vi "Логи_Флаги.vi"() -> ()   [LabVIEW 2013]
panel:
  in  "Tab Control":T1(tab)
  out "?":cluster{dbl[], u16[]}[](graph)
  out "XY":cluster{dbl[], dbl[]}[](graph)
  out "double precision float":dbl
  out "ID параметров":u8[](array[numeric])
  out "Заголовок":string
  out "Количество параметров":u8
  out "size (in bytes)":i64
  # "1-VALUE_TRANSMITTED\n2-VOLTAGE_LOW\n3-FAIL_SENSOR\t\n4-ARMING_DISARMING\n5-FLAG_FAIL_SD\n6-FLAG_LIFT_COMMAND"
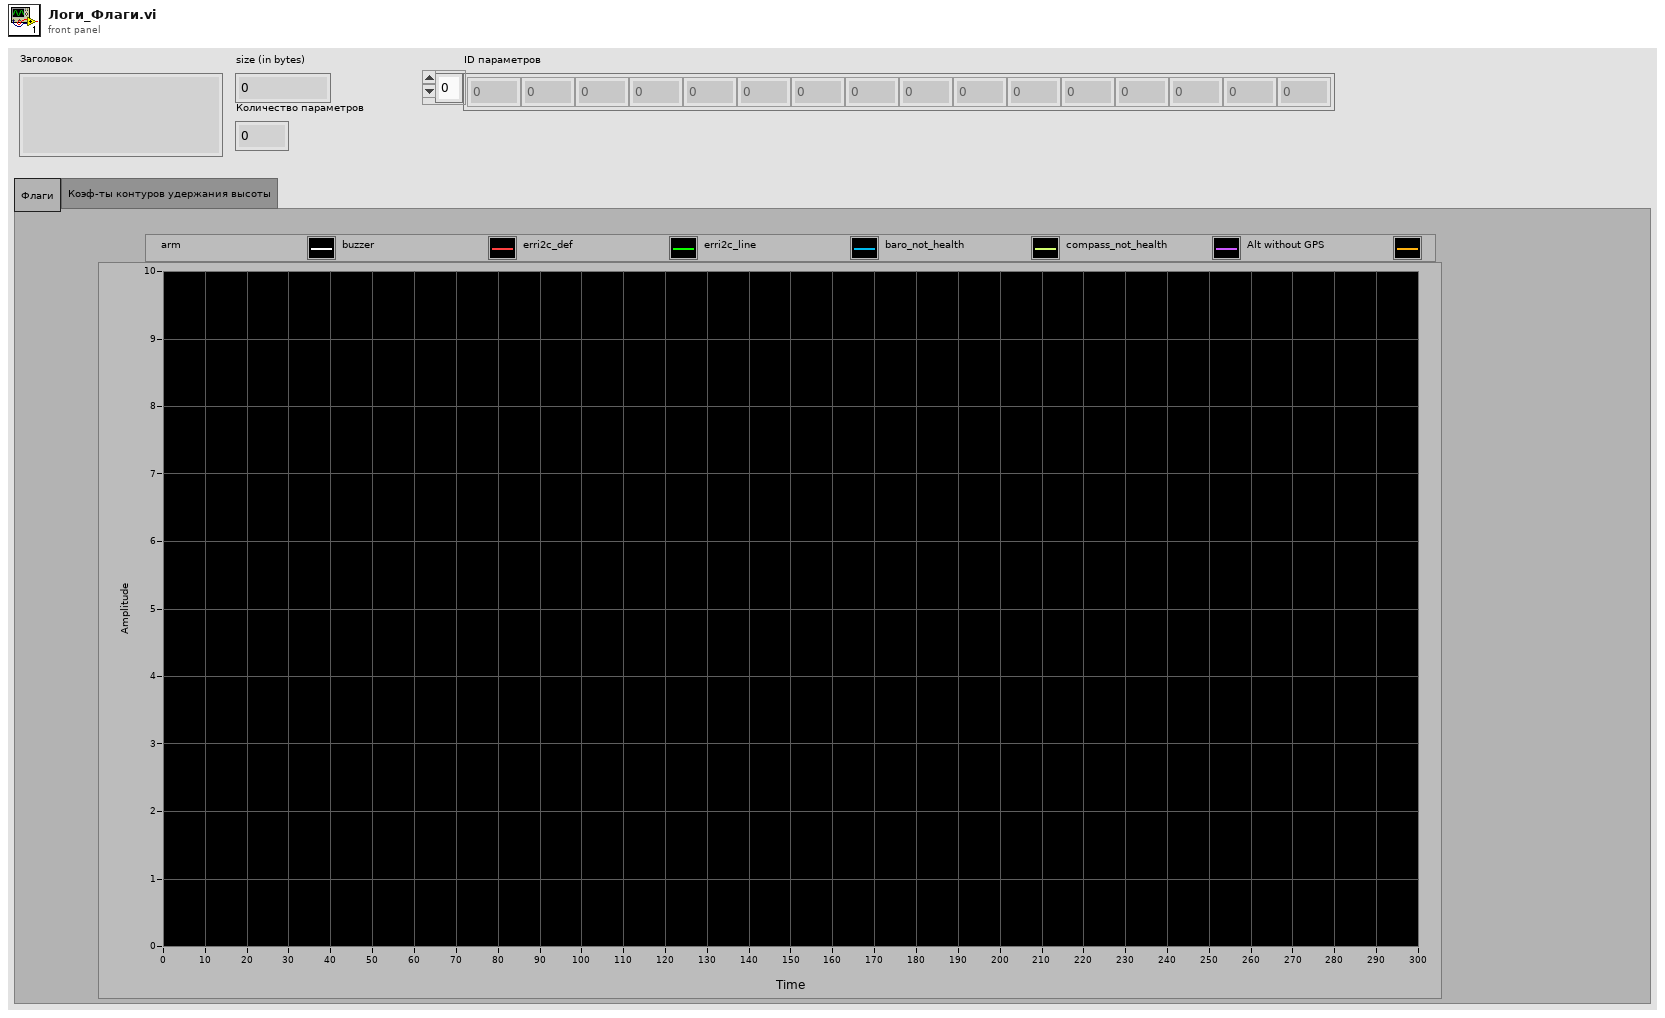
[diagram p1: front panel]
types:
  T1 = enum32{"Флаги", "Коэф-ты контуров удержания высоты"}
  T2 = enum16{"open", "replace", "create", "open or create", "replace or create", "replace or create with confirmation"}
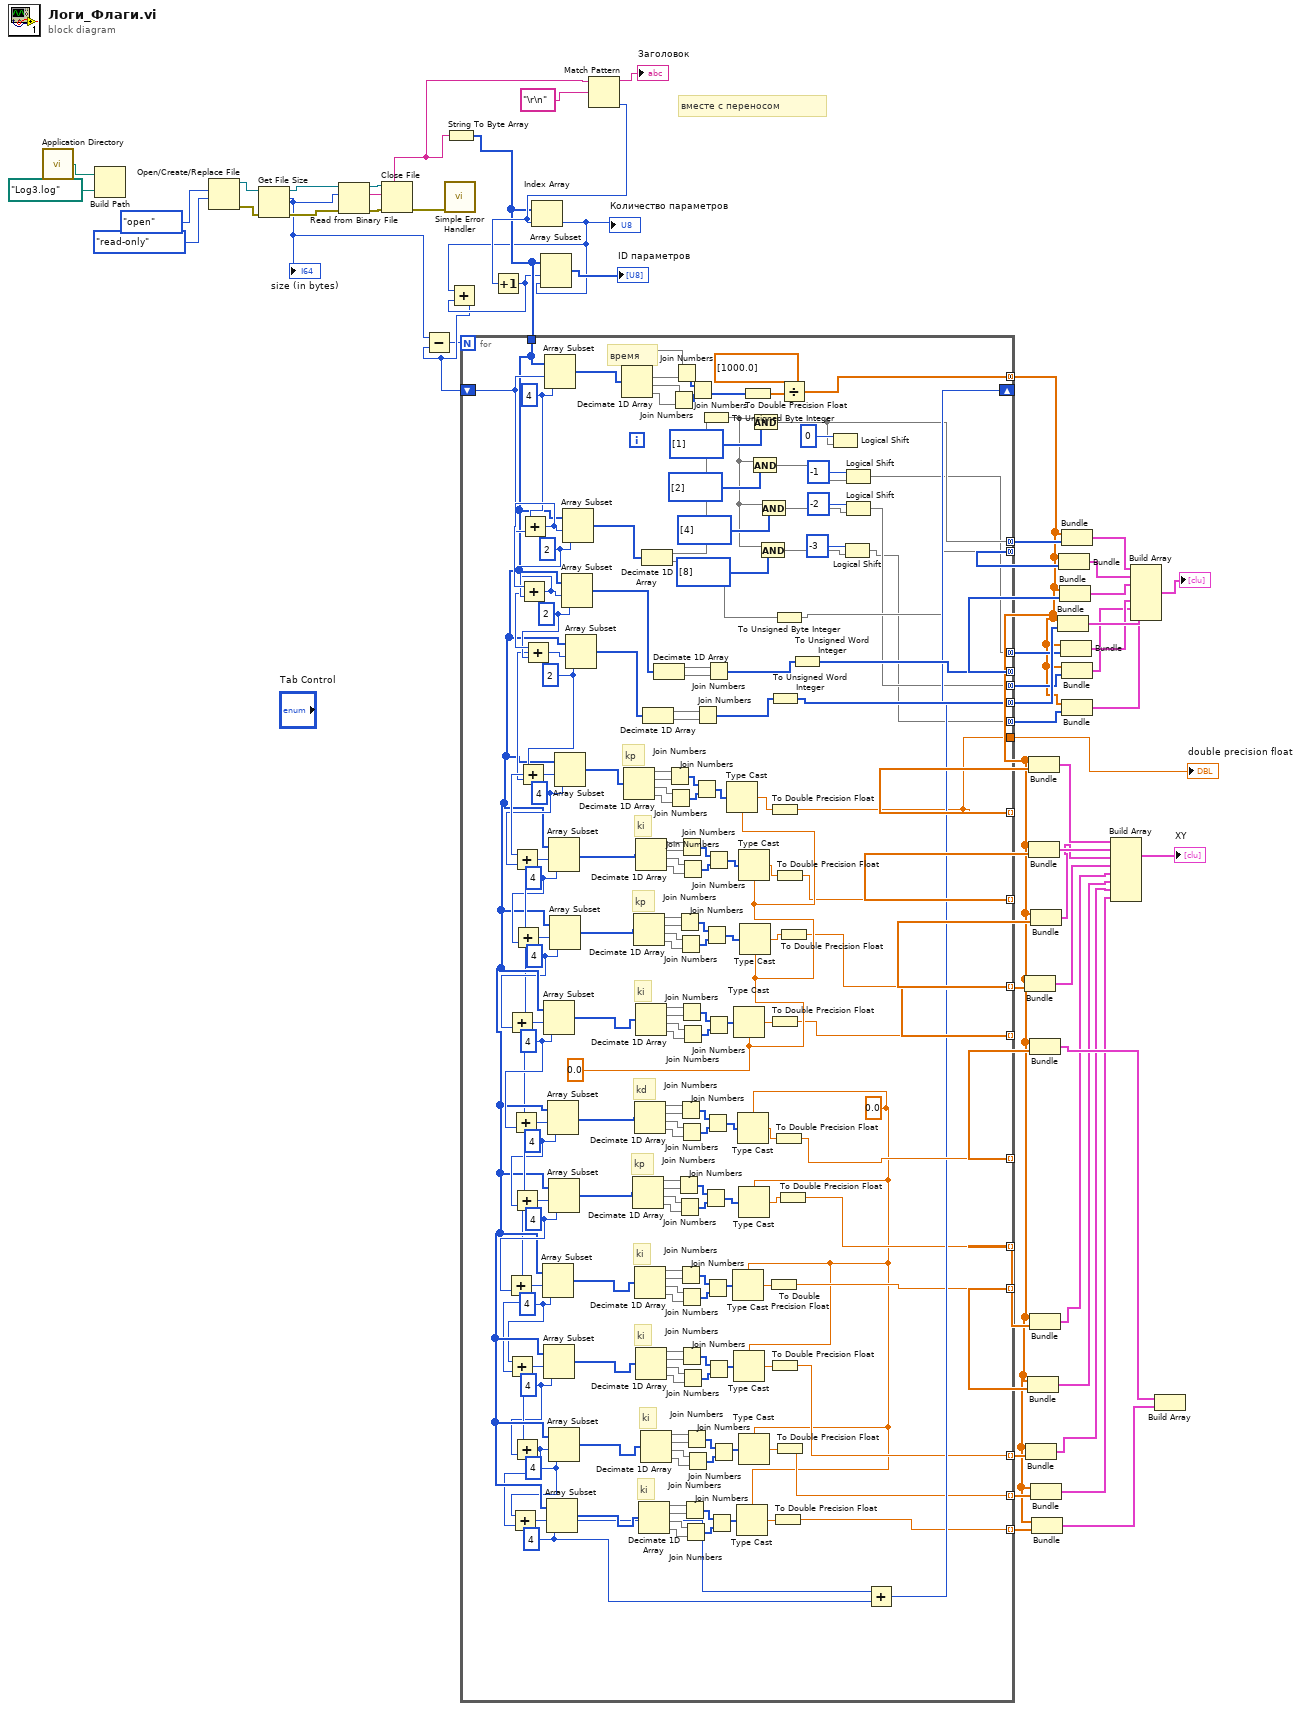
[diagram p0: block diagram]
diagram:
  # "вместе с переносом"
  n1 = call <vilib>:"Application Directory.vi"() -> ("Application Directory"=w57:path)
  n2 = Build Path(base path=w57, name or relative path=path "Log3.log" ("default name")) -> ()  [unwired: 1 out]
  n3 = Open/Create/Replace File(operation (0:open)=T2."open", access (0:read/write)=enum16{"read/write", "read-only", "write-only"}."read-only") -> (refnum out=w54:refnum<file>, error out=w52:errorcluster)  [unwired: 4 in, 1 out]
  n4 = Get File Size(file=w54, error in=w52) -> (refnum out=w53:refnum<file>, size (in bytes)=w44:i64, 0:w51:errorcluster)
  "size (in bytes)" <- w44
  n5 = Read from Binary File(8:w51, 10:w44, 11:w53) -> (0:w55:errorcluster, 2:w50:string, 3:w56:refnum<file>)  [unwired: 3 in, 1 out]
  n6 = Close File(refnum=w56, error in=w55) -> (error out=w60:errorcluster)  [unwired: 1 out]
  n7 = call <vilib>:"Simple Error Handler.vi"("error in (no error)"=w60) -> ()  [unwired: 4 in, 5 out]
  n8 = String To Byte Array(string=w50) -> (unsigned byte array=w45:u8[])
  n9 = Match Pattern(string=w50, regular expression="\r\n" ("format string")) -> (before substring=→"Заголовок":string, offset past match=w47:i32)  [unwired: 1 in, 2 out]
  n10 = Increment(x=w47) -> (x+1=w42:i32)
  n11 = Index Array(array=w45, index=w47) -> (element=w43:u8)
  "Количество параметров" <- w43
  n12 = Add(x=w43, y=w42) -> (x+y=w41:i32)
  n13 = Subtract(x=w44, y=w41) -> (x-y=w40:i64)
  n14 = for {
    N: w40 -> [_]
    tunnel: w45 -> [w95]
    shift-right: [w132] -> _
    shift-left: w41 -> [w125]
    tunnel: [w78] -> w39 mode=indexing
    tunnel: [w180] -> w37 mode=indexing
    tunnel: [w181] -> w38 mode=indexing
    tunnel: [w182] -> w36 mode=indexing
    tunnel: [w166] -> w28 mode=concatenating
    tunnel: [w168] -> w27 mode=concatenating
    tunnel: [w133] -> w22 mode=indexing
    tunnel: [w131] -> w21 mode=indexing
    tunnel: [w130] -> w20 mode=indexing
    tunnel: [w128] -> w3 mode=concatenating
    tunnel: [w127] -> w29 mode=concatenating
    tunnel: [w82] -> w19 mode=indexing
    tunnel: [w81] -> w17 mode=indexing
    tunnel: [w80] -> w16 mode=indexing
    tunnel: [w78] -> w15
    tunnel: [w72] -> w9 mode=concatenating
    tunnel: [w67] -> w5 mode=concatenating
    tunnel: [w66] -> w4 mode=concatenating
    tunnel: [w61] -> w2 mode=concatenating
    w91 = 4 ("length")
    w90 = 4 ("length")
    w87 = 4 ("length")
    w79 = sgl 0.0
    w86 = 4 ("length")
    w164 = 4 ("length")
    w162 = 4 ("length")
    w124 = 2 ("length")
    w169 = 2 ("length")
    w171 = 2 ("length")
    w185 = sgl 0.0
    w134 = 4 ("length")
    w94 = 4 ("length")
    w230 = 4 ("length")
    w232 = 4 ("length")
    w126 = 4 ("length")
    # "ki"
    # "ki"
    # "ki"
    # "ki"
    # "kp"
    # "kd"
    # "ki"
    # "kp"
    # "ki"
    # "kp"
    # "время"
    n15 = Add(x=w126, y=w125) -> (x+y=w172:i32)
    n16 = Add(x=w172, y=w171) -> (x+y=w170:i32)
    n17 = Add(x=w170, y=w169) -> (x+y=w123:i32)
    n18 = Add(x=w124, y=w123) -> (x+y=w233:i32)
    n19 = Add(x=w233, y=w232) -> (x+y=w231:i32)
    n20 = Add(x=w231, y=w230) -> (x+y=w93:i32)
    n21 = Add(x=w93, y=w94) -> (x+y=w83:i32)
    n22 = Add(x=w83, y=w134) -> (x+y=w163:i32)
    n23 = Add(x=w163, y=w162) -> (x+y=w84:i32)
    n24 = Add(x=w84, y=w164) -> (x+y=w85:i32)
    n25 = Add(x=w86, y=w85) -> (x+y=w88:i32)
    n26 = Add(x=w88, y=w87) -> (x+y=w89:i32)
    n27 = Add(x=w90, y=w89) -> (x+y=w92:i32)
    n28 = Array Subset(array=w95, index=w85, length=w86) -> (w141:u8[])
    n29 = Array Subset(array=w95, index=w83, length=w134) -> (w193:u8[])
    n30 = Array Subset(array=w95, index=w88, length=w87) -> (w116:u8[])
    n31 = Array Subset(array=w95, index=w125, length=w126) -> (w220:u8[])
    n32 = Array Subset(array=w95, index=w92, length=w91) -> (w98:u8[])
    n33 = Array Subset(array=w95, index=w163, length=w162) -> (w155:u8[])
    n34 = Array Subset(array=w95, index=w231, length=w230) -> (w207:u8[])
    n35 = Array Subset(array=w95, index=w84, length=w164) -> (w148:u8[])
    n36 = Array Subset(array=w95, index=w89, length=w90) -> (w107:u8[])
    n37 = Array Subset(array=w95, index=w93, length=w94) -> (w200:u8[])
    n38 = Array Subset(array=w95, index=w233, length=w232) -> (w221:u8[])
    n39 = Array Subset(array=w95, index=w170, length=w169) -> (w176:u8[])
    n40 = Array Subset(array=w95, index=w172, length=w171) -> (w179:u8[])
    n41 = Array Subset(array=w95, index=w123, length=w124) -> (w173:u8[])
    n42 = Decimate 1D Array(w220) -> (w223:u8[], w224:u8[], w225:u8[], w226:u8[])
    n43 = Decimate 1D Array(w221) -> (w228:u8[], w229:u8[], w217:u8[], w216:u8[])
    n44 = Decimate 1D Array(w148) -> (w153:u8[], w154:u8[], w152:u8[], w151:u8[])
    n45 = Decimate 1D Array(w200) -> (w205:u8[], w206:u8[], w204:u8[], w203:u8[])
    n46 = Decimate 1D Array(w155) -> (w160:u8[], w161:u8[], w159:u8[], w158:u8[])
    n47 = Decimate 1D Array(w141) -> (w146:u8[], w147:u8[], w145:u8[], w144:u8[])
    n48 = Decimate 1D Array(w207) -> (w212:u8[], w213:u8[], w211:u8[], w210:u8[])
    n49 = Decimate 1D Array(w193) -> (w198:u8[], w199:u8[], w197:u8[], w196:u8[])
    n50 = Decimate 1D Array(w116) -> (w121:u8[], w122:u8[], w120:u8[], w119:u8[])
    n51 = Decimate 1D Array(w98) -> (w103:u8[], w104:u8[], w102:u8[], w101:u8[])
    n52 = Decimate 1D Array(w107) -> (w112:u8[], w113:u8[], w111:u8[], w110:u8[])
    n53 = Decimate 1D Array(w179) -> (w76:u8[], w129:u8[])
    n54 = Decimate 1D Array(w173) -> (w174:u8[], w175:u8[])
    n55 = Decimate 1D Array(w176) -> (w177:u8[], w178:u8[])
    n56 = Join Numbers(hi=w228, lo=w229) -> ((hi.lo)=w215:u16[])
    n57 = Join Numbers(hi=w217, lo=w216) -> ((hi.lo)=w214:u16[])
    n58 = Join Numbers(hi=w225, lo=w226) -> ((hi.lo)=w222:u16[])
    n59 = Join Numbers(hi=w223, lo=w224) -> ((hi.lo)=w227:u16[])
    n60 = Join Numbers(hi=w153, lo=w154) -> ((hi.lo)=w150:u16[])
    n61 = Join Numbers(hi=w205, lo=w206) -> ((hi.lo)=w202:u16[])
    n62 = Join Numbers(hi=w152, lo=w151) -> ((hi.lo)=w149:u16[])
    n63 = Join Numbers(hi=w204, lo=w203) -> ((hi.lo)=w201:u16[])
    n64 = Join Numbers(hi=w160, lo=w161) -> ((hi.lo)=w157:u16[])
    n65 = Join Numbers(hi=w146, lo=w147) -> ((hi.lo)=w143:u16[])
    n66 = Join Numbers(hi=w212, lo=w213) -> ((hi.lo)=w209:u16[])
    n67 = Join Numbers(hi=w198, lo=w199) -> ((hi.lo)=w195:u16[])
    n68 = Join Numbers(hi=w159, lo=w158) -> ((hi.lo)=w156:u16[])
    n69 = Join Numbers(hi=w145, lo=w144) -> ((hi.lo)=w142:u16[])
    n70 = Join Numbers(hi=w121, lo=w122) -> ((hi.lo)=w118:u16[])
    n71 = Join Numbers(hi=w211, lo=w210) -> ((hi.lo)=w208:u16[])
    n72 = Join Numbers(hi=w197, lo=w196) -> ((hi.lo)=w194:u16[])
    n73 = Join Numbers(hi=w120, lo=w119) -> ((hi.lo)=w117:u16[])
    n74 = Join Numbers(hi=w103, lo=w104) -> ((hi.lo)=w100:u16[])
    n75 = Join Numbers(hi=w102, lo=w101) -> ((hi.lo)=w99:u16[])
    n76 = Join Numbers(hi=w112, lo=w113) -> ((hi.lo)=w109:u16[])
    n77 = Join Numbers(hi=w111, lo=w110) -> ((hi.lo)=w108:u16[])
    n78 = Join Numbers(hi=w227, lo=w222) -> ((hi.lo)=w188:u32[])
    n79 = Join Numbers(hi=w215, lo=w214) -> ((hi.lo)=w184:u32[])
    n80 = Join Numbers(hi=w174, lo=w175) -> ((hi.lo)=w167:u16[])
    n81 = To Unsigned Byte Integer(number=w76) -> (unsigned 8bit integer=w62:u8[])
    n82 = Join Numbers(hi=w150, lo=w149) -> ((hi.lo)=w138:u32[])
    n83 = Join Numbers(hi=w202, lo=w201) -> ((hi.lo)=w190:u32[])
    n84 = Join Numbers(hi=w157, lo=w156) -> ((hi.lo)=w136:u32[])
    n85 = Join Numbers(hi=w143, lo=w142) -> ((hi.lo)=w139:u32[])
    n86 = Join Numbers(hi=w177, lo=w178) -> ((hi.lo)=w165:u16[])
    n87 = Join Numbers(hi=w209, lo=w208) -> ((hi.lo)=w187:u32[])
    n88 = Join Numbers(hi=w195, lo=w194) -> ((hi.lo)=w191:u32[])
    n89 = Join Numbers(hi=w118, lo=w117) -> ((hi.lo)=w114:u32[])
    n90 = Join Numbers(hi=w100, lo=w99) -> ((hi.lo)=w96:u32[])
    n91 = Join Numbers(hi=w109, lo=w108) -> ((hi.lo)=w105:u32[])
    n92 = Type Cast(type=w185, x=w184) -> (*(type *) &x=w183:sgl)
    n93 = Type Cast(type=w79, x=w139) -> (*(type *) &x=w140:sgl)
    n94 = Type Cast(type=w185, x=w191) -> (*(type *) &x=w192:sgl)
    n95 = Type Cast(type=w79, x=w114) -> (*(type *) &x=w115:sgl)
    n96 = Type Cast(type=w79, x=w96) -> (*(type *) &x=w97:sgl)
    n97 = Type Cast(type=w79, x=w136) -> (*(type *) &x=w135:sgl)
    n98 = Type Cast(type=w185, x=w187) -> (*(type *) &x=w186:sgl)
    n99 = Type Cast(type=w79, x=w138) -> (*(type *) &x=w137:sgl)
    n100 = Type Cast(type=w79, x=w105) -> (*(type *) &x=w106:sgl)
    n101 = Type Cast(type=w185, x=w190) -> (*(type *) &x=w189:sgl)
    n102 = To Double Precision Float(number=w188) -> (double precision float=w219:dbl[])
    n103 = And(x=w62, y=u8[] [2]) -> (x .and. y?=w71:u8[])
    n104 = And(x=w62, y=u8[] [1]) -> (x .and. y?=w72:u8[])
    n105 = And(x=w62, y=u8[] [8]) -> (x .and. y?=w64:u8[])
    n106 = And(x=w62, y=u8[] [4]) -> (x .and. y?=w69:u8[])
    n107 = To Double Precision Float(number=w140) -> (double precision float=w130:dbl)
    n108 = To Unsigned Word Integer(number=w167) -> (unsigned 16bit integer=w168:u16[])
    n109 = To Double Precision Float(number=w183) -> (double precision float=w78:dbl)
    n110 = To Double Precision Float(number=w192) -> (double precision float=w182:dbl)
    n111 = To Double Precision Float(number=w115) -> (double precision float=w82:dbl)
    n112 = To Double Precision Float(number=w97) -> (double precision float=w80:dbl)
    n113 = To Unsigned Byte Integer(number=w129) -> (unsigned 8bit integer=w127:u8[])
    n114 = To Double Precision Float(number=w135) -> (double precision float=w133:dbl)
    n115 = To Double Precision Float(number=w186) -> (double precision float=w180:dbl)
    n116 = To Double Precision Float(number=w106) -> (double precision float=w81:dbl)
    n117 = To Double Precision Float(number=w137) -> (double precision float=w131:dbl)
    n118 = Divide(x=w219, y=dbl[] [1000.0]) -> (x/y=w128:dbl[])
    n119 = To Double Precision Float(number=w189) -> (double precision float=w181:dbl)
    n120 = To Unsigned Word Integer(number=w165) -> (unsigned 16bit integer=w166:u16[])
    n121 = Logical Shift(y=i16 0, x=w72) -> ()  [unwired: 1 out]
    n122 = Logical Shift(y=i16 -3, x=w64) -> (x << y=w61:u8[])
    n123 = Logical Shift(y=i16 -1, x=w71) -> (x << y=w67:u8[])
    n124 = Logical Shift(y=i16 -2, x=w69) -> (x << y=w66:u8[])
    n125 = Add(x=w92, y=w91) -> (x+y=w132:i32)
  }
  "double precision float" <- w15
  n126 = Array Subset(array=w45, index=w42, length=w43) -> (→"ID параметров":u8[])
  n127 = Bundle(w3, w36) -> (w32:cluster{dbl[], dbl[]})  [unwired: 1 in]
  n128 = Bundle(w3, w19) -> (w11:cluster{dbl[], dbl[]})  [unwired: 1 in]
  n129 = Bundle(w3, w20) -> (w12:cluster{dbl[], dbl[]})  [unwired: 1 in]
  n130 = Bundle(w3, w39) -> (w35:cluster{dbl[], dbl[]})  [unwired: 1 in]
  n131 = Bundle(w3, w37) -> (w34:cluster{dbl[], dbl[]})  [unwired: 1 in]
  n132 = Bundle(w3, w22) -> (w14:cluster{dbl[], dbl[]})  [unwired: 1 in]
  n133 = Bundle(w3, w21) -> (w13:cluster{dbl[], dbl[]})  [unwired: 1 in]
  n134 = Bundle(w3, w38) -> (w33:cluster{dbl[], dbl[]})  [unwired: 1 in]
  n135 = Bundle(w3, w17) -> (w10:cluster{dbl[], dbl[]})  [unwired: 1 in]
  n136 = Bundle(w3, w16) -> (w18:cluster{dbl[], dbl[]})  [unwired: 1 in]
  n137 = Bundle(w3, w27) -> (w24:cluster{dbl[], u16[]})  [unwired: 1 in]
  n138 = Bundle(w3, w29) -> (w26:cluster{dbl[], u8[]})  [unwired: 1 in]
  n139 = Bundle(w3, w28) -> (w25:cluster{dbl[], u16[]})  [unwired: 1 in]
  n140 = Bundle(w3, w5) -> (w7:cluster{dbl[], u8[]})  [unwired: 1 in]
  n141 = Bundle(w3, w9) -> (w8:cluster{dbl[], u8[]})  [unwired: 1 in]
  n142 = Bundle(w3, w4) -> (w6:cluster{dbl[], u8[]})  [unwired: 1 in]
  n143 = Bundle(w3, w2) -> (w1:cluster{dbl[], u8[]})  [unwired: 1 in]
  n144 = Build Array(w35, w34, w33, w32, w13, w12, w11, w10) -> (→"XY":cluster{dbl[], dbl[]}[])
  n145 = Build Array(w8, w26, w25, w24, w7, w6, w1) -> (→"?":cluster{dbl[], u16[]}[])
  n146 = Build Array(w14, w18) -> ()  [unwired: 1 out]
